vi "Create Serial Input Channel I2C IO x4.vi"() -> (4 "serial input channel i2c io x4":T2)   [LabVIEW 2023, in "GettingStarted_Common_148X_FPGA.lvlib"]
uses:
  GettingStarted_Common_148X_FPGA.lvlib
  Types/I2C IO.ctl
  <instrlib>/_niInstr/Basic Elements/v1/FPGA/niInstr Basic Elements v1 FPGA.lvlib
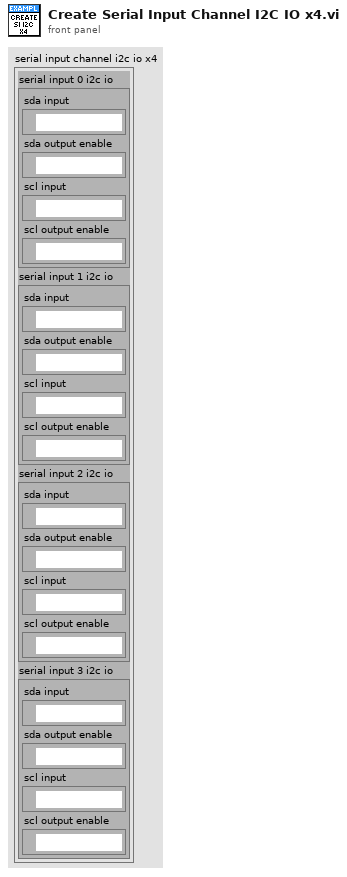
[diagram p1: front panel]
types:
  T1 = typedef "GettingStarted_Common_148X_FPGA.lvlib/I2C IO.ctl" = cluster{"sda input":refnum<k21>, "sda output enable":refnum<k21>, "scl input":refnum<k21>, "scl output enable":refnum<k21>}
  T2 = cluster{"serial input 0 i2c io":T1, "serial input 1 i2c io":T1, "serial input 2 i2c io":T1, "serial input 3 i2c io":T1}
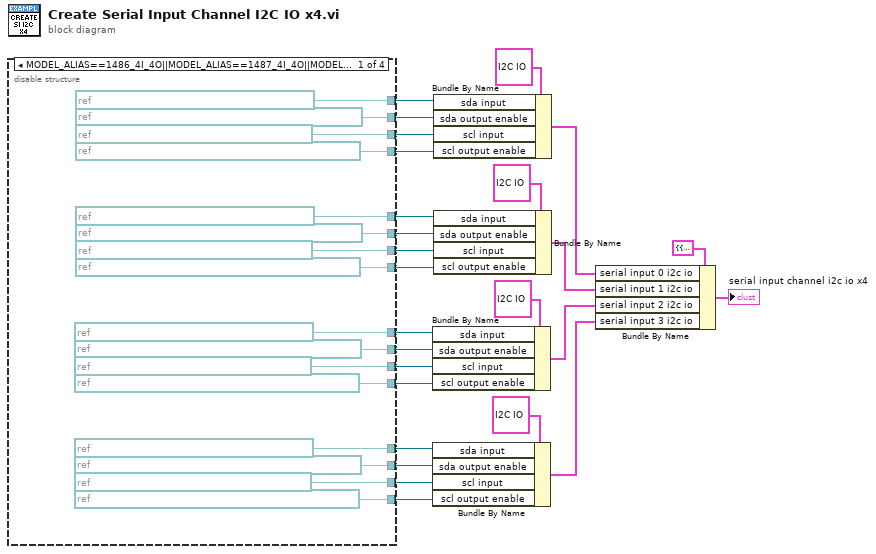
[diagram p0: block diagram]
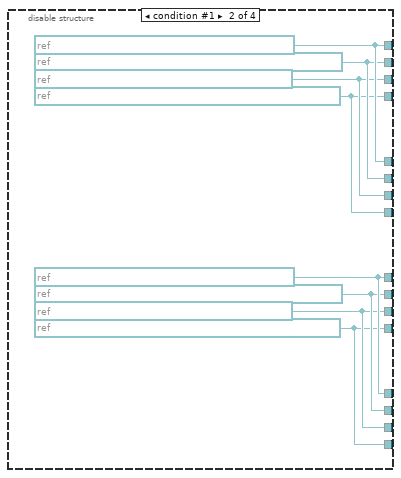
[diagram p2: hidden frame]
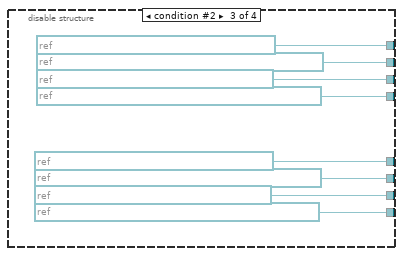
[diagram p3: hidden frame]
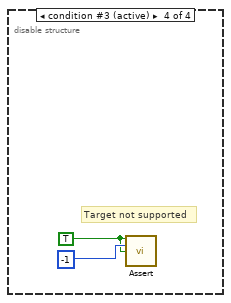
[diagram p4: hidden frame]
diagram:
  n1 = disable-structure shown="MODEL_ALIAS==1486_4I_4O||MODEL_ALIAS==1487_4I_4O||MODEL_ALIAS==1488_4I_4O" {
    disable-tunnel: [refnum<k21> "IO Socket\\SI 2 Deserializer I2C SCL Output Enable" ("scl output enable") w43 _ _] -> w11
    disable-tunnel: [refnum<k21> "IO Socket\\SI 2 Deserializer I2C SCL Input" ("scl input") w44 _ _] -> w12
    disable-tunnel: [refnum<k21> "IO Socket\\SI 2 Deserializer I2C SDA Output Enable" ("sda output enable") w45 _ _] -> w13
    disable-tunnel: [refnum<k21> "IO Socket\\SI 2 Deserializer I2C SDA Input" ("sda input") w46 _ _] -> w14
    disable-tunnel: [refnum<k21> "IO Socket\\SI 3 Deserializer I2C SDA Input" ("sda input") w46 _ _] -> w10
    disable-tunnel: [refnum<k21> "IO Socket\\SI 3 Deserializer I2C SDA Output Enable" ("sda output enable") w45 _ _] -> w9
    disable-tunnel: [refnum<k21> "IO Socket\\SI 3 Deserializer I2C SCL Input" ("scl input") w44 _ _] -> w8
    disable-tunnel: [refnum<k21> "IO Socket\\SI 3 Deserializer I2C SCL Output Enable" ("scl output enable") w43 _ _] -> w7
    disable-tunnel: [refnum<k21> "IO Socket\\SI 1 Deserializer I2C SCL Output Enable" ("scl output enable") w47 refnum<k21> "IO Socket\\SI 1 Deserializer I2C SCL Output Enable" ("scl output enable") _] -> w15
    disable-tunnel: [refnum<k21> "IO Socket\\SI 1 Deserializer I2C SCL Input" ("scl input") w48 refnum<k21> "IO Socket\\SI 1 Deserializer I2C SCL Input" ("scl input") _] -> w16
    disable-tunnel: [refnum<k21> "IO Socket\\SI 1 Deserializer I2C SDA Output Enable" ("sda output enable") w49 refnum<k21> "IO Socket\\SI 1 Deserializer I2C SDA Output Enable" ("sda output enable") _] -> w17
    disable-tunnel: [refnum<k21> "IO Socket\\SI 1 Deserializer I2C SDA Input" ("sda input") w50 refnum<k21> "IO Socket\\SI 1 Deserializer I2C SDA Input" ("sda input") _] -> w18
    disable-tunnel: [refnum<k21> "IO Socket\\SI 0 Deserializer I2C SDA Input" ("sda input") w50 refnum<k21> "IO Socket\\SI 0 Deserializer I2C SDA Input" ("sda input") _] -> w22
    disable-tunnel: [refnum<k21> "IO Socket\\SI 0 Deserializer I2C SDA Output Enable" ("sda output enable") w49 refnum<k21> "IO Socket\\SI 0 Deserializer I2C SDA Output Enable" ("sda output enable") _] -> w19
    disable-tunnel: [refnum<k21> "IO Socket\\SI 0 Deserializer I2C SCL Input" ("scl input") w48 refnum<k21> "IO Socket\\SI 0 Deserializer I2C SCL Input" ("scl input") _] -> w20
    disable-tunnel: [refnum<k21> "IO Socket\\SI 0 Deserializer I2C SCL Output Enable" ("scl output enable") w47 refnum<k21> "IO Socket\\SI 0 Deserializer I2C SCL Output Enable" ("scl output enable") _] -> w21
    frame condition #0 {
    }
    frame condition #1 {
      w43 = refnum<k21> "IO Socket\\SI 2 SI 3 Deserializer I2C SCL Output Enable" ("scl output enable")
      w44 = refnum<k21> "IO Socket\\SI 2 SI 3 Deserializer I2C SCL Input" ("scl input")
      w45 = refnum<k21> "IO Socket\\SI 2 SI 3 Deserializer I2C SDA Output Enable" ("sda output enable")
      w46 = refnum<k21> "IO Socket\\SI 2 SI 3 Deserializer I2C SDA Input" ("sda input")
      w47 = refnum<k21> "IO Socket\\SI 0 SI 1 Deserializer I2C SCL Output Enable" ("scl output enable")
      w48 = refnum<k21> "IO Socket\\SI 0 SI 1 Deserializer I2C SCL Input" ("scl input")
      w49 = refnum<k21> "IO Socket\\SI 0 SI 1 Deserializer I2C SDA Output Enable" ("sda output enable")
      w50 = refnum<k21> "IO Socket\\SI 0 SI 1 Deserializer I2C SDA Input" ("sda input")
    }
    frame condition #2 {
    }
    frame condition #3 (active) {
      w59 = TRUE ("assert")
      # "Target not supported"
      n2 = call <instrlib>:"Assert.vi"("assert"=w59, "error code"=-1, "enable show error"=w59) -> ()  [unwired: 13 in]
    }
  }
  n3 = Bundle By Name(cluster=T1 {"sda input"="IO Socket\\SI 0 Deserializer I2C SDA Input", "sda output enable"="IO Socket\\SI 0 Deserializer I2C SDA Output Enable", "scl input"="IO Socket\\SI 0 Deserializer I2C SCL Input", "scl output enable"="IO Socket\\SI 0 Deserializer I2C SCL Output Enable"}, "sda input"=w14, "sda output enable"=w13, "scl input"=w12, "scl output enable"=w11) -> (w3:T1)
  n4 = Bundle By Name(cluster=T1 {"sda input"="IO Socket\\SI 0 Deserializer I2C SDA Input", "sda output enable"="IO Socket\\SI 0 Deserializer I2C SDA Output Enable", "scl input"="IO Socket\\SI 0 Deserializer I2C SCL Input", "scl output enable"="IO Socket\\SI 0 Deserializer I2C SCL Output Enable"}, "sda input"=w10, "sda output enable"=w9, "scl input"=w8, "scl output enable"=w7) -> (w2:T1)
  n5 = Bundle By Name(cluster=T1 {"sda input"="IO Socket\\SI 0 Deserializer I2C SDA Input", "sda output enable"="IO Socket\\SI 0 Deserializer I2C SDA Output Enable", "scl input"="IO Socket\\SI 0 Deserializer I2C SCL Input", "scl output enable"="IO Socket\\SI 0 Deserializer I2C SCL Output Enable"}, "sda input"=w22, "sda output enable"=w19, "scl input"=w20, "scl output enable"=w21) -> (w5:T1)
  n6 = Bundle By Name(cluster=T1 {"sda input"="IO Socket\\SI 0 Deserializer I2C SDA Input", "sda output enable"="IO Socket\\SI 0 Deserializer I2C SDA Output Enable", "scl input"="IO Socket\\SI 0 Deserializer I2C SCL Input", "scl output enable"="IO Socket\\SI 0 Deserializer I2C SCL Output Enable"}, "sda input"=w18, "sda output enable"=w17, "scl input"=w16, "scl output enable"=w15) -> (w4:T1)
  n7 = Bundle By Name(cluster=T2 {"serial input 0 i2c io"={"sda input"="IO Socket\\SI 0 Deserializer I2C SDA Input", "sda output enable"="IO Socket\\SI 0 Deserializer I2C SDA Output Enable", "scl input"="IO Socket\\SI 0 Deserializer I2C SCL Input", "scl output enable"="IO Socket\\SI 0 Deserializer I2C SCL Output Enable"}, "serial input 1 i2c io"={"sda input"="IO Socket\\SI 0 Deserializer I2C SDA Input", "sda output enable"="IO Socket\\SI 0 Deserializer I2C SDA Output Enable", "scl input"="IO Socket\\SI 0 Deserializer I2C SCL Input", "scl output enable"="IO Socket\\SI 0 Deserializer I2C SCL Output Enable"}, "serial input 2 i2c io"={"sda input"="IO Socket\\SI 0 Deserializer I2C SDA Input", "sda output enable"="IO Socket\\SI 0 Deserializer I2C SDA Output Enable", "scl input"="IO Socket\\SI 0 Deserializer I2C SCL Input", "scl output enable"="IO Socket\\SI 0 Deserializer I2C SCL Output Enable"}, "serial input 3 i2c io"={"sda input"="IO Socket\\SI 0 Deserializer I2C SDA Input", "sda output enable"="IO Socket\\SI 0 Deserializer I2C SDA Output Enable", "scl input"="IO Socket\\SI 0 Deserializer I2C SCL Input", "scl output enable"="IO Socket\\SI 0 Deserializer I2C SCL Output Enable"}} ("serial input channel i2c io x4"), "serial input 0 i2c io"=w5, "serial input 1 i2c io"=w4, "serial input 2 i2c io"=w3, "serial input 3 i2c io"=w2) -> (→"serial input channel i2c io x4":T2)
